vi "Read Timeout.vi"(8 "error in (no error)":errorcluster, 11 "Client in":refnum<class "CV-Client.lvclass">) -> (0 "error out":errorcluster, 2 "Send timeout":i32 caption="Send timeout [ms]", 3 "Client out":refnum<class "CV-Client.lvclass">)   [LabVIEW 2013, in "CameraVision.lvlib" / "CV-Client.lvclass"]
uses:
  CV-Client.lvclass
  CV-Client.lvclass/CV-Client.ctl
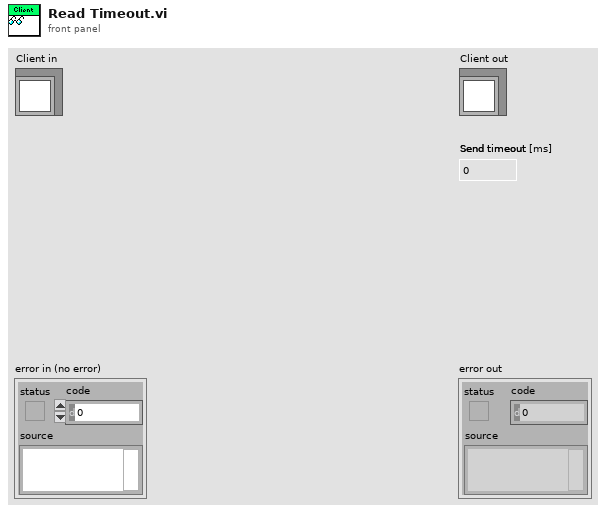
[diagram p1: front panel]
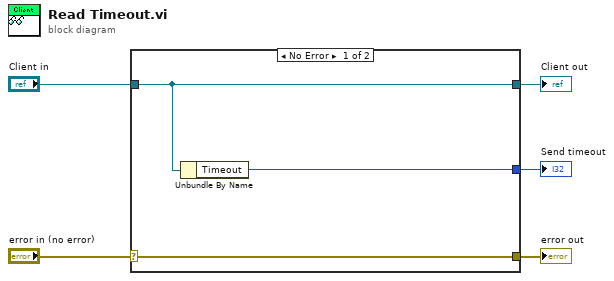
[diagram p0: block diagram]
diagram:
  n1 = case shown="No Error" "error in (no error)" {
    selector: "error in (no error)" -> [w8 w9]
    tunnel: [w8 w9] -> w4
    tunnel: [w7 w10] -> w2
    tunnel: "Client in" -> [w7 w10]
    tunnel: [w6 _] -> w1
    frame No Error {
      n2 = Unbundle By Name(w7) -> ("Timeout"=w6:i32)
    }
    frame Error {
    }
  }
  "error out" <- w4
  "Client out" <- w2
  "Send timeout" <- w1
